vi "Write Languages.vi"(8 "error in (no error)":errorcluster, 10 "Languages []":T1[](array[typedef]), 11 "ResFile in":refnum<class "Resource Data.lvclass">) -> (0 "error out":errorcluster, 3 "ResFile out":refnum<class "Resource Data.lvclass">)   [LabVIEW 2013, in "SET Project Data.lvlib" / "Resource Data.lvclass"]
uses:
  Resource Data.lvclass
  Types/ProjFile_Language Entry.ctl
  Resource Data.lvclass/Resource Data.ctl
  SET Project Data.lvlib
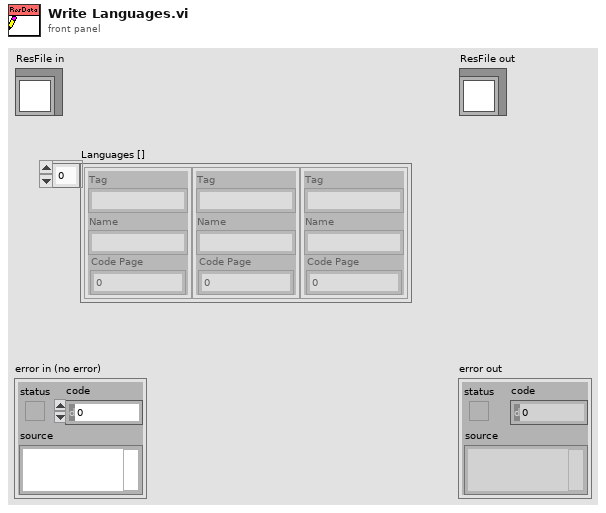
[diagram p1: front panel]
types:
  T1 = typedef "SET Project Data.lvlib/ProjFile_Language Entry.ctl" = cluster{"Tag":string, "Name":string, "Code Page":u16}
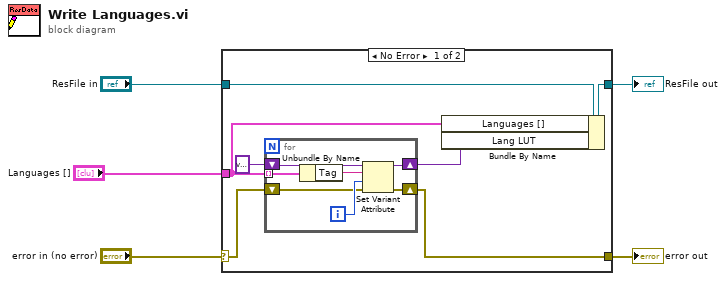
[diagram p0: block diagram]
diagram:
  n1 = case shown="No Error" "error in (no error)" {
    selector: "error in (no error)" -> [w8 w20]
    tunnel: [w7 w20] -> w4
    tunnel: [w11 w21] -> w2
    tunnel: "ResFile in" -> [w12 w21]
    tunnel: "Languages []" -> [w6 _]
    frame No Error {
      n2 = for {
        shift-right: [w18] -> w9
        shift-left: variant ("variant") -> [w19]
        tunnel: w6 -> [w14] mode=indexing
        shift-right: [w15] -> w7
        shift-left: w8 -> [w16]
        i -> [w17]
        n3 = Unbundle By Name(w14) -> ("Tag"=w13:string)
        n4 = Set Variant Attribute(Variant=w19, name=w13, value=w17, error in=w16) -> (Variant out=w18:variant, error out=w15:errorcluster)  [unwired: 1 out]
      }
      n5 = Bundle By Name(cluster=w12, "Languages []"=w6, "Lang LUT"=w9) -> (w11:refnum<class "Resource Data.lvclass">)
    }
    frame Error {
    }
  }
  "error out" <- w4
  "ResFile out" <- w2
